vi "Xsens RotMatrix(SubVI).vi"(1 "DATA in (Hex)":string) -> (0 "Rot Matrix":T1)   [LabVIEW 2019]
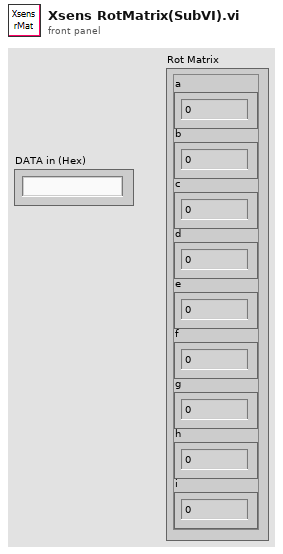
[diagram p1: front panel]
types:
  T1 = cluster{"a":sgl, "b":sgl, "c":sgl, "d":sgl, "e":sgl, "f":sgl, "g":sgl, "h":sgl, "i":sgl}
  T2 = cluster{sgl, sgl, sgl, sgl, sgl, sgl, sgl, sgl, sgl}
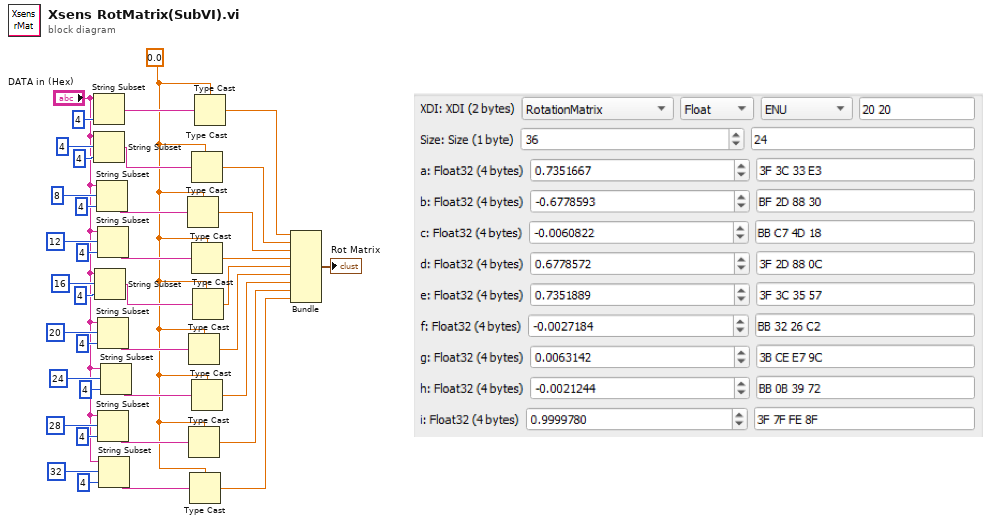
[diagram p0: block diagram]
diagram:
  w8 = sgl 0.0
  n1 = String Subset(string="DATA in (Hex)", length (rest)=4 ("length (rest)")) -> (substring=w34:string)  [unwired: 1 in]
  n2 = String Subset(string="DATA in (Hex)", offset (0)=4, length (rest)=4 ("length (rest)")) -> (substring=w29:string)
  n3 = String Subset(string="DATA in (Hex)", offset (0)=16, length (rest)=4 ("length (rest)")) -> (substring=w19:string)
  n4 = String Subset(string="DATA in (Hex)", offset (0)=8, length (rest)=4 ("length (rest)")) -> (substring=w28:string)
  n5 = String Subset(string="DATA in (Hex)", offset (0)=12, length (rest)=4 ("length (rest)")) -> (substring=w25:string)
  n6 = String Subset(string="DATA in (Hex)", offset (0)=20, length (rest)=4 ("length (rest)")) -> (substring=w18:string)
  n7 = String Subset(string="DATA in (Hex)", offset (0)=28, length (rest)=4 ("length (rest)")) -> (substring=w12:string)
  n8 = String Subset(string="DATA in (Hex)", offset (0)=32, length (rest)=4 ("length (rest)")) -> (substring=w9:string)
  n9 = String Subset(string="DATA in (Hex)", offset (0)=24, length (rest)=4 ("length (rest)")) -> (substring=w15:string)
  n10 = Type Cast(type=w8, x=w28) -> (*(type *) &x=w36:sgl)
  n11 = Type Cast(type=w8, x=w18) -> (*(type *) &x=w5:sgl)
  n12 = Type Cast(type=w8, x=w12) -> (*(type *) &x=w3:sgl)
  n13 = Type Cast(type=w8, x=w9) -> (*(type *) &x=w2:sgl)
  n14 = Type Cast(type=w8, x=w29) -> (*(type *) &x=w37:sgl)
  n15 = Type Cast(type=w8, x=w25) -> (*(type *) &x=w24:sgl)
  n16 = Type Cast(type=w8, x=w15) -> (*(type *) &x=w4:sgl)
  n17 = Type Cast(type=w8, x=w19) -> (*(type *) &x=w6:sgl)
  n18 = Type Cast(type=w8, x=w34) -> (*(type *) &x=w38:sgl)
  n19 = Bundle(w38, w37, w36, w24, w6, w5, w4, w3, w2) -> (→"Rot Matrix":T2)  [unwired: 1 in]
